vi "Convert Shutdown Furnace to Heater State Enum-setup.vi"(11 "test case ID":string) -> (3 "Shutdown Furnace":bool)   [LabVIEW 2018]
doc: "The setup VI should be executed before the VI under test in the harness VI. In this VI you can prepare the environment and the inputs of the VI under test.\n\nSee the Help Document for more information. (<b>Help</b> > <b>IncQuery Labs</b> > <b>InstaCoverage</b> > <b>InstaCoverage Help...</b>)"
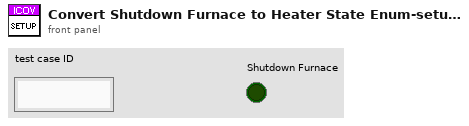
[diagram p1: front panel]
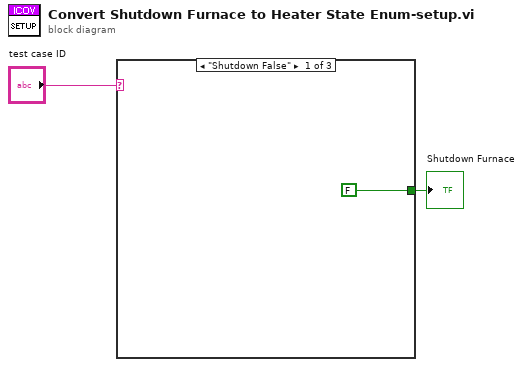
[diagram p0: block diagram]
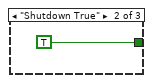
[diagram p2: hidden frame]
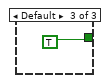
[diagram p3: hidden frame]
diagram:
  n1 = case shown="\"Shutdown False\"" "test case ID" {
    tunnel: [FALSE TRUE TRUE] -> w1
    frame "Shutdown False" {
    }
    frame "Shutdown True" {
    }
    frame Default {
    }
  }
  "Shutdown Furnace" <- w1
